vi "PlotBG Draw.vi"(7 "scale locked?":T2, 8 "error in (no error)":errorcluster, 11 "Draw Area Size":T1) -> (0 "error out":errorcluster, 3 "picture":picture)   [LabVIEW 2021, in "RocketPlot.lvlib"]
uses:
  RocketPlot.lvlib
  TypeDefs/plotBG inputs.ctl
  <vilib>/Utility/miscctls.llb/LVBoundsTypeDef.ctl
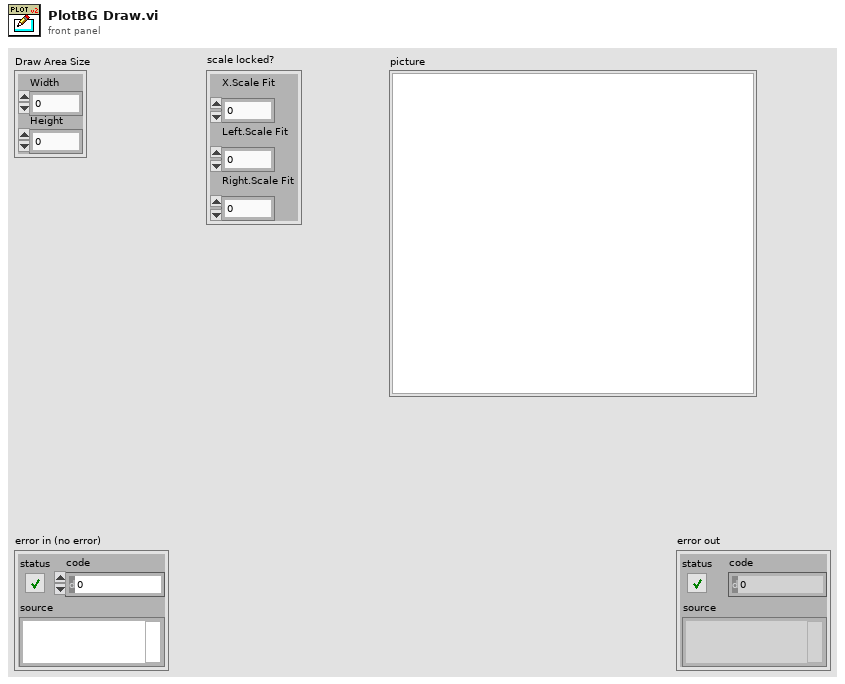
[diagram p1: front panel]
types:
  T1 = typedef "LVBoundsTypeDef.ctl" = cluster{"Width":u32, "Height":u32}
  T2 = typedef "RocketPlot.lvlib/plotBG inputs.ctl" = cluster{"X.Scale Fit":u8, "Left.Scale Fit":u8, "Right.Scale Fit":u8}
  T3 = cluster{"Width":i16, "Style":enum32{"Solid", "Dash", "Dot", "DashDot", "DashDotDot"}}
  T4 = cluster{"left":i16, "top":i16, "right":i16, "bottom":i16}
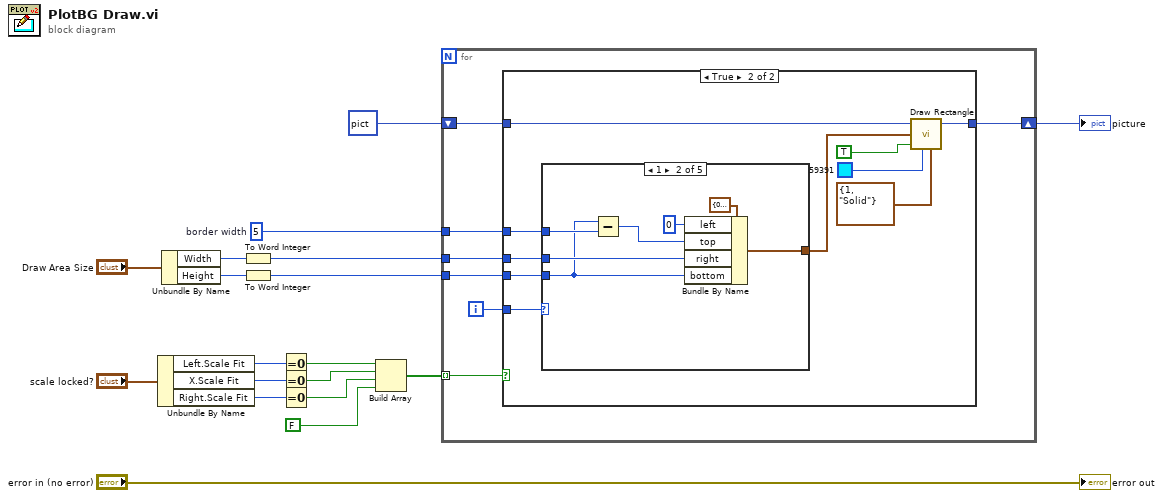
[diagram p0: block diagram]
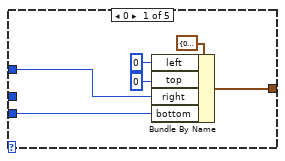
[diagram p3: hidden frame]
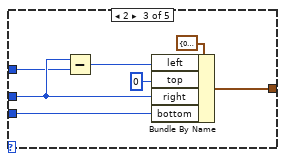
[diagram p4: hidden frame]
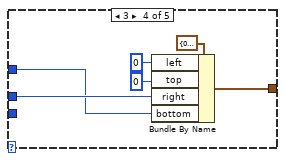
[diagram p5: hidden frame]
diagram:
  w1 = i16 5  # border width
  n1 = Unbundle By Name("scale locked?") -> ("Left.Scale Fit"=w10:u8, "X.Scale Fit"=w8:u8, "Right.Scale Fit"=w7:u8)
  n2 = Unbundle By Name("Draw Area Size") -> ("Width"=w18:u32, "Height"=w17:u32)
  n3 = To Word Integer(number=w18) -> (16bit integer=w15:i16)
  n4 = To Word Integer(number=w17) -> (16bit integer=w14:i16)
  n5 = Equal To 0?(x=w10) -> (x = 0?=w9:bool)
  n6 = Equal To 0?(x=w8) -> (x = 0?=w6:bool)
  n7 = Equal To 0?(x=w7) -> (x = 0?=w5:bool)
  n8 = Build Array(w9, w6, w5, FALSE ("element")) -> (w11:bool[])
  n9 = for {
    shift-right: [w21] -> w4
    shift-left: picture data[5B] ("picture") -> [w22]
    tunnel: w15 -> [w25]
    tunnel: w14 -> [w24]
    tunnel: w11 -> [w20] mode=indexing
    tunnel: w1 -> [w19]
    i -> [w23]
    n10 = case shown="True" w20 {
      tunnel: w25 -> [_ w36]
      tunnel: w24 -> [_ w35]
      tunnel: w23 -> [_ w34]
      tunnel: w22 -> [w26 w33]
      tunnel: [w26 w32] -> w21
      tunnel: w19 -> [_ w27]
      frame False {
      }
      frame True {
        n11 = case shown="1" w34 {
          tunnel: w36 -> [_ w46 w52 w59 _]
          tunnel: w35 -> [w38 w43 w53 _ _]
          tunnel: [w39 w48 w55 w61 _] -> w31
          tunnel: w27 -> [w37 w45 w51 w57 _]
          frame 0 {
            n12 = Bundle By Name(cluster=T4 {"left"=0, "top"=0, "right"=0, "bottom"=0} ("rect"), "left"=i16 0, "top"=i16 0, "right"=w37, "bottom"=w38) -> (w39:T4)
          }
          frame 1 {
            n13 = Subtract(x=w43, y=w45) -> (x-y=w44:i16)
            n14 = Bundle By Name(cluster=T4 {"left"=0, "top"=0, "right"=0, "bottom"=0} ("rect"), "left"=i16 0, "top"=w44, "right"=w46, "bottom"=w43) -> (w48:T4)
          }
          frame 2 {
            n15 = Subtract(x=w52, y=w51) -> (x-y=w50:i16)
            n16 = Bundle By Name(cluster=T4 {"left"=0, "top"=0, "right"=0, "bottom"=0} ("rect"), "left"=w50, "top"=i16 0, "right"=w52, "bottom"=w53) -> (w55:T4)
          }
          frame 3 {
            n17 = Bundle By Name(cluster=T4 {"left"=0, "top"=0, "right"=0, "bottom"=0} ("rect"), "left"=i16 0, "top"=i16 0, "right"=w59, "bottom"=w57) -> (w61:T4)
          }
          frame Default {
          }
        }
        n18 = call <vilib>:"Draw Rectangle.vi"("picture"=w33, "rect"=w31, "fill?(F)"=TRUE, "color(black)"=u32 59391, "pen"=T3 {"Width"=1, "Style"=enum."Solid"}) -> ("new picture"=w32:picture)  [unwired: 4 in]
      }
    }
  }
  "picture" <- w4
  "error out" <- "error in (no error)"
